vi "Add Step to Measurement Sequence.vi"(8 "error in (no error)":errorcluster, 10 "Step to Add":refnum<k7>, 11 "Measurement Interface in":refnum<class "Measurement Interface.lvclass">) -> (0 "error out":errorcluster, 3 "Measurement Interface out":refnum<class "Measurement Interface.lvclass">)   [LabVIEW 2016, in "Measurement Interface.lvlib" / "Measurement Interface.lvclass"]
uses:
  Measurement Interface.lvclass
  Measurement Interface.lvclass/Measurement Interface.ctl
  Plugins/TestStand API Tools (TSAT).lvlibp/Sequence Actions/TSAT Sequence Actions.lvlib
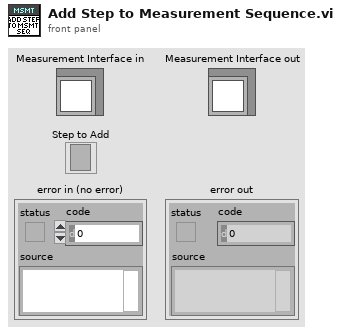
[diagram p1: front panel]
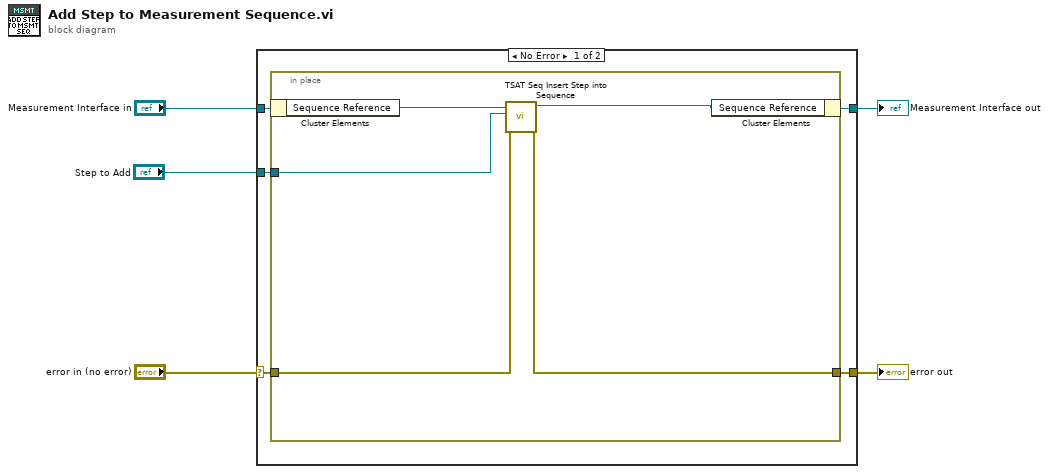
[diagram p0: block diagram]
diagram:
  n1 = case shown="No Error" "error in (no error)" {
    selector: "error in (no error)" -> [w9 w17]
    tunnel: [w8 w17] -> w4
    tunnel: [w6 w16] -> w2
    tunnel: "Measurement Interface in" -> [w10 w16]
    tunnel: "Step to Add" -> [w7 _]
    frame No Error {
      n2 = in-place {
        in-place-border: w9 -> [w13]
        in-place-border: [w12] -> w8
        in-place-border: w7 -> [w11]
        n3 = in-place-cluster #1(w10) -> ("Sequence Reference"=w15:refnum<k7>)
        n4 = call "TSAT Seq Insert Step into Sequence.vi"("Error in"=w13, "Step to Add"=w11, "Sequence In"=w15) -> ("error out"=w12:errorcluster, "Sequence Out"=w14:refnum<k7>)  [unwired: 7 in]
        n5 = in-place-cluster #1("Sequence Reference"=w14) -> (w6:refnum<class "Measurement Interface.lvclass">)
      }
    }
    frame Error {
    }
  }
  "error out" <- w4
  "Measurement Interface out" <- w2
